vi "HW operation 2.vi"(1 "Combo Box":string(combo), 2 "Numeric":dbl) -> (0 "Numeric 2":dbl, 3 "Numeric 3":dbl)   [LabVIEW 2017]
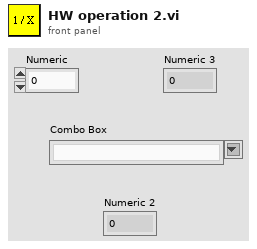
[diagram p1: front panel]
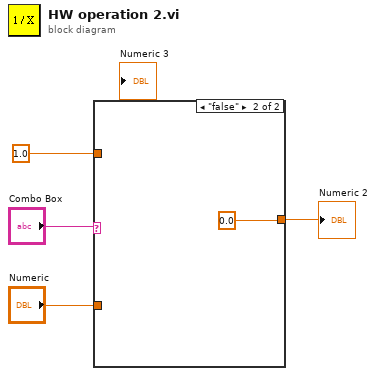
[diagram p0: block diagram]
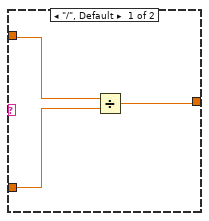
[diagram p2: hidden frame]
diagram:
  n1 = case shown="\"false\"" "Combo Box" {
    tunnel: "Numeric" -> [w5 _]
    tunnel: 1.0 -> [w6 _]
    tunnel: [w7 0.0] -> w1
    frame "/", Default {
      n2 = Divide(x=w6, y=w5) -> (x/y=w7:dbl)
    }
    frame "false" {
    }
  }
  "Numeric 2" <- w1
